vi "Check VI Version.vi"(0 "lab view version":string, 5 "vi path":path, 11 "error in":errorcluster) -> (4 "incompatible version warning":string, 15 "error out":errorcluster)   [LabVIEW 2021, in "Converter.lvlib"]
uses:
  Converter.lvlib
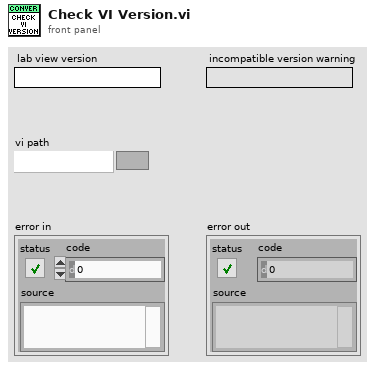
[diagram p1: front panel]
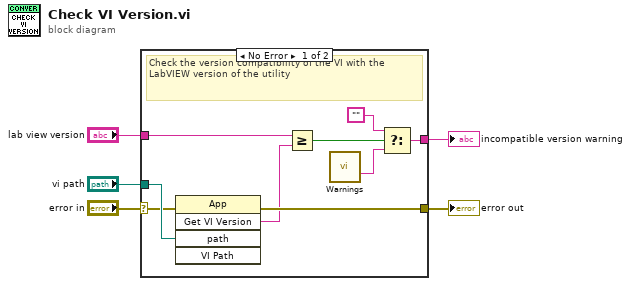
[diagram p0: block diagram]
diagram:
  n1 = case shown="No Error" "error in" {
    selector: "error in" -> [w6 w15]
    tunnel: [w14 w15] -> w5
    tunnel: [w13 _] -> w4
    tunnel: "lab view version" -> [w9 _]
    tunnel: "vi path" -> [w7 _]
    frame No Error {
      # "Check the version compatibility of the VI with the LabVIEW version of the utility"
      n2 = invoke class="App" method="Get VI Version"(error in=w6, "path"=w7) -> (error out=w14:errorcluster, "GetVIVers"=w8:string)  [unwired: 3 in, 3 out]
      n3 = Greater Or Equal?(x=w9, y=w8) -> (x >= y?=w10:bool)
      n4 = call "Warnings.vi"() -> ("incompatible measurement version"=w12:string)  [unwired: 8 in, 7 out]
      n5 = Select(t="", s=w10, f=w12) -> (s? t:f=w13:string)
    }
    frame Error {
      # "Pass"
    }
  }
  "error out" <- w5
  "incompatible version warning" <- w4
